vi "Unit to Point.vi"(3 "X unit":sgl, 4 "Unit (default = mm)":T1=enum."mm") -> (9 "X point":sgl)   [LabVIEW 2013]
uses:
  Controls/Unit.ctl
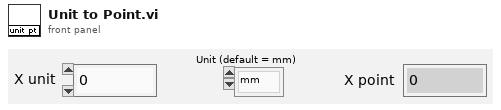
[diagram p1: front panel]
types:
  T1 = typedef "Unit.ctl" = enum16{"inch", "mm"}
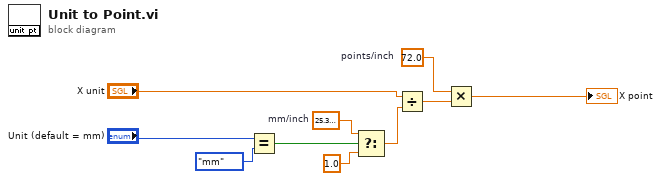
[diagram p0: block diagram]
diagram:
  w3 = sgl 25.4  # mm/inch
  w9 = sgl 72.0  # points/inch
  n1 = Equal?(x="Unit (default = mm)", y=Unit."mm") -> (x = y?=w4:bool)
  n2 = Select(t=w3, s=w4, f=sgl 1.0) -> (s? t:f=w2:sgl)
  n3 = Divide(x="X unit", y=w2) -> (x/y=w10:sgl)
  n4 = Multiply(x=w9, y=w10) -> (x*y=→"X point":sgl)
